vi "BS1200 Discovery - Get Tag Value.vi"(9 "Name":string, 10 "Initial Filter":string, 11 "Input String":string) -> (3 "Value":string)   [LabVIEW 2021, in "BS120x Driver.lvlib"]
uses:
  BS120x Driver.lvlib
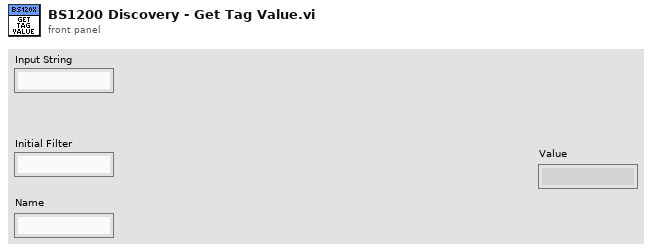
[diagram p1: front panel]
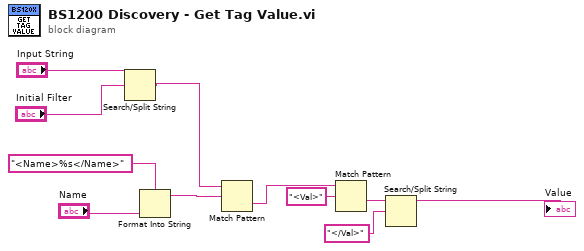
[diagram p0: block diagram]
diagram:
  n1 = Search/Split String(string="Input String", search string/char (-)="Initial Filter") -> (match + rest of string=w1:string)  [unwired: 1 in, 2 out]
  n2 = Format Into String(format string="<Name>%s</Name>", "Name") -> (resulting string=w5:string)  [unwired: 2 in, 1 out]
  n3 = Match Pattern(string=w1, regular expression=w5) -> (after substring=w10:string)  [unwired: 1 in, 3 out]
  n4 = Match Pattern(string=w10, regular expression="<Val>") -> (after substring=w8:string)  [unwired: 1 in, 3 out]
  n5 = Search/Split String(string=w8, search string/char (-)="</Val>" ("input")) -> (substring before match=→"Value":string)  [unwired: 1 in, 2 out]
